vi "per socket shutdown.vi"(8 "error in (no error)":errorcluster, 11 "Websocket console plugin in":refnum<class "Websocket console plugin.lvclass">) -> (0 "error out":errorcluster)   [LabVIEW 2013, in "Websocket console plugin.lvclass"]
uses:
  Websocket console plugin.lvclass
  websocket user plugin.lvclass
  Websocket console plugin.lvclass/Websocket console plugin.ctl
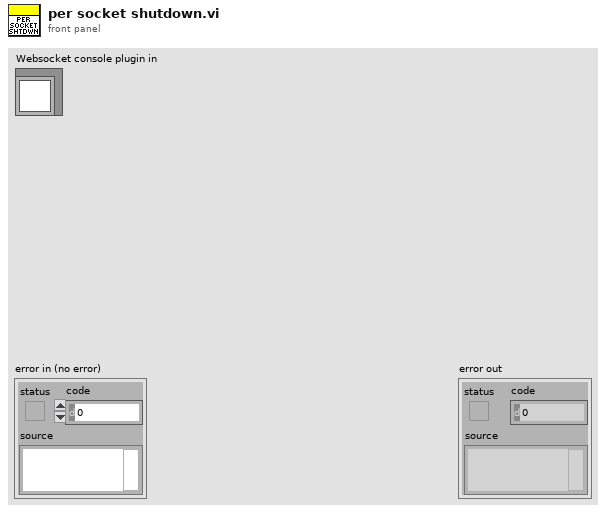
[diagram p1: front panel]
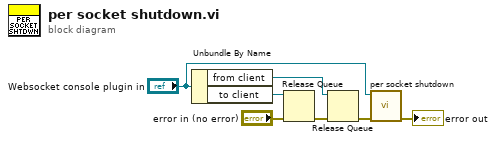
[diagram p0: block diagram]
diagram:
  n1 = Unbundle By Name("Websocket console plugin in") -> ("from client"=w1:refnum<queue>, "to client"=w2:refnum<queue>)
  n2 = Release Queue(queue=w2, error in (no error)="error in (no error)") -> (error out=w4:errorcluster)  [unwired: 1 in, 2 out]
  n3 = Release Queue(queue=w1, error in (no error)=w4) -> (error out=w3:errorcluster)  [unwired: 1 in, 2 out]
  n4 = call-parent "per socket shutdown.vi"("error in (no error)"=w3, "websocket user plugin in"="Websocket console plugin in") -> ("error out"=→"error out":errorcluster)  [unwired: 9 in]
